vi "init.vi"(8 "error in":errorcluster, 10 "TBM module configuration in":refnum<class "TBM module configuration.lvclass">, 11 "bin datalogger runtime in":refnum<class "Binary datalogger runtime.lvclass">) -> (0 "error out":errorcluster, 1 "data allocations":T1, 2 "execution settings":T4, 3 "bin datalogger runtime out":refnum<class "Binary datalogger runtime.lvclass">)   [LabVIEW 2013, in "Binary datalogger runtime.lvclass"]
doc: "Provides an interface for initializing a module at runtime. While this interface performs no operations, a child should provide an override which may open any necessary references or sessions, allocate necessary memory, and perform any final configuration validataion before providing the full configuration <b>execution data</b> to the calling process."
uses:
  Binary datalogger runtime.lvclass
  <vilib>/NI/Tag Bus Module Framework/channel/TBM channel.lvclass
  <vilib>/NI/Tag Bus Module Framework/runtime/TBM module execution interface.lvclass
  configuration/Binary datalogger configuration.lvclass
  <vilib>/NI/Tag Bus Module Framework/runtime/execution settings.ctl
  control enum.ctl
  <vilib>/NI/Tag Bus/table/data table.ctl
  <vilib>/NI/Tag Bus/table/data table.lvlib
  <vilib>/NI/Tag Bus/dictionary/data dictionary.lvclass
  message to background process.ctl
  response enum.ctl
  response from background process.ctl
  <vilib>/NI/Tag Bus Module Framework/module configuration/TBM module configuration.lvclass
  <vilib>/NI/Tag Bus Module Framework/channel/data tables.ctl
  <vilib>/NI/Tag Bus/dictionary table pair.ctl
  <vilib>/NI/Tag Bus/tag bus.lvlib
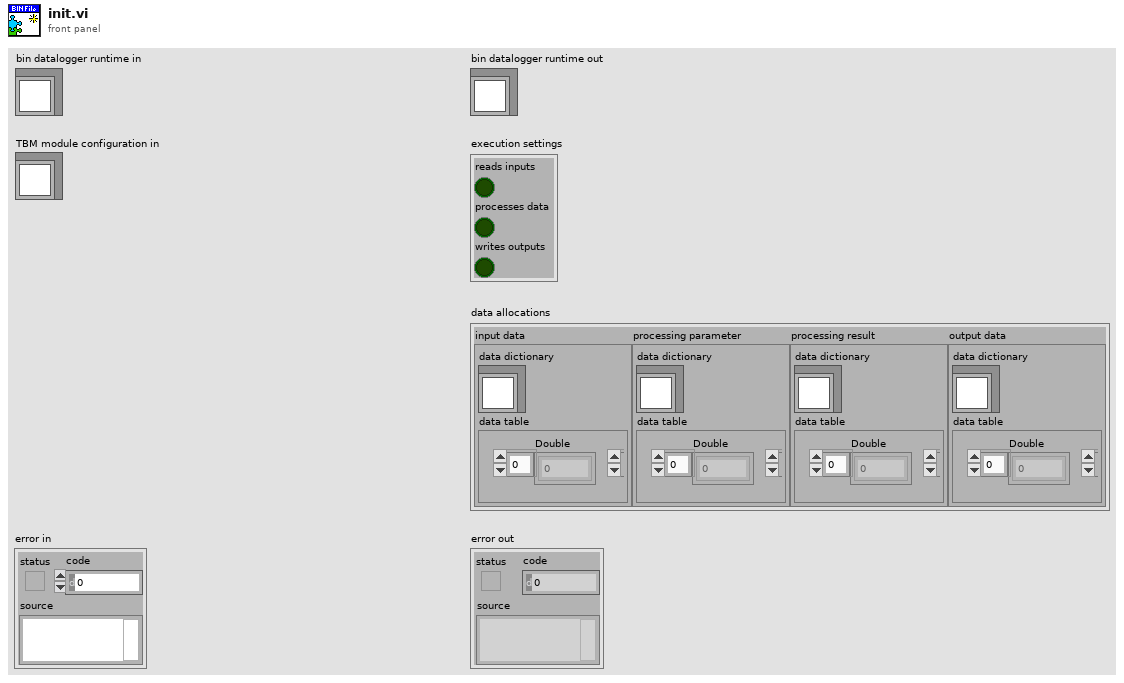
[diagram p1: front panel]
types:
  T1 = typedef "TBM channel.lvclass/data tables.ctl" = cluster{"input data":T2, "processing parameter":T2, "processing result":T2, "output data":T2}
  T2 = typedef "tag bus.lvlib/dictionary table pair.ctl" = cluster{"data dictionary":refnum<class "data dictionary.lvclass">, "data table":T3}
  T3 = typedef "tag bus.lvlib/data table.lvlib/data table.ctl" = cluster{"Double":dbl[], "Single":sgl[], "I64":i64[], "I32":i32[], "I16":i16[], "I8":i8[], "U64":u64[], "U32":u32[], "U16":u16[], "U8":u8[], "Boolean":bool[], "String":string[], "Array of Double":cluster{"DBL Array":dbl[]}[], "Array of Single":cluster{"SGL Array":sgl[]}[], "Array of I64":cluster{"I64 Array":i64[]}[], "Array of I32":cluster{"I32 Array":i32[]}[], "Array of I16":cluster{"I16 Array":i16[]}[], "Array of I8":cluster{"I8 Array":i8[]}[], "Array of U64":cluster{"U64 Array":u64[]}[], "Array of U32":cluster{"U32 Array":u32[]}[], "Array of U16":cluster{"U16 Array":u16[]}[], "Array of U8":cluster{"U8 Array":u8[]}[], "Array of Boolean":cluster{"Boolean Array":bool[]}[], "Array of String":cluster{"String Array":string[]}[]}
  T4 = typedef "TBM module execution interface.lvclass/execution settings.ctl" = cluster{"reads inputs":bool, "processes data":bool, "writes outputs":bool}
  T5 = cluster{"read mode":enum16{"polling", "blocking"}, "write mode":enum16{"polling", "blocking"}}
  T6 = typedef "Binary datalogger runtime.lvclass/response from background process.ctl" = cluster{"response enum":T7, "datapack":refnum<data-value>, "error code":i32}
  T7 = typedef "Binary datalogger runtime.lvclass/response enum.ctl" = enum16{"exit", "return buffer", "error"}
  T8 = typedef "Binary datalogger runtime.lvclass/message to background process.ctl" = cluster{"control enum":T9, "datapack":refnum<data-value>, "Time Stamp":timestamp}
  T9 = typedef "Binary datalogger runtime.lvclass/control enum.ctl" = enum16{"exit", "output data"}
  T10 = typedef "tag bus.lvlib/data dictionary.lvclass/full data dictionary.ctl" = cluster{"Double":string[], "Single":string[], "I64":string[], "I32":string[], "I16":string[], "I8":string[], "U64":string[], "U32":string[], "U16":string[], "U8":string[], "Boolean":string[], "String":string[], "Array of Double":string[], "Array of Single":string[], "Array of I64":string[], "Array of I32":string[], "Array of I16":string[], "Array of I8":string[], "Array of U64":string[], "Array of U32":string[], "Array of U16":string[], "Array of U8":string[], "Array of Boolean":string[], "Array of String":string[]}
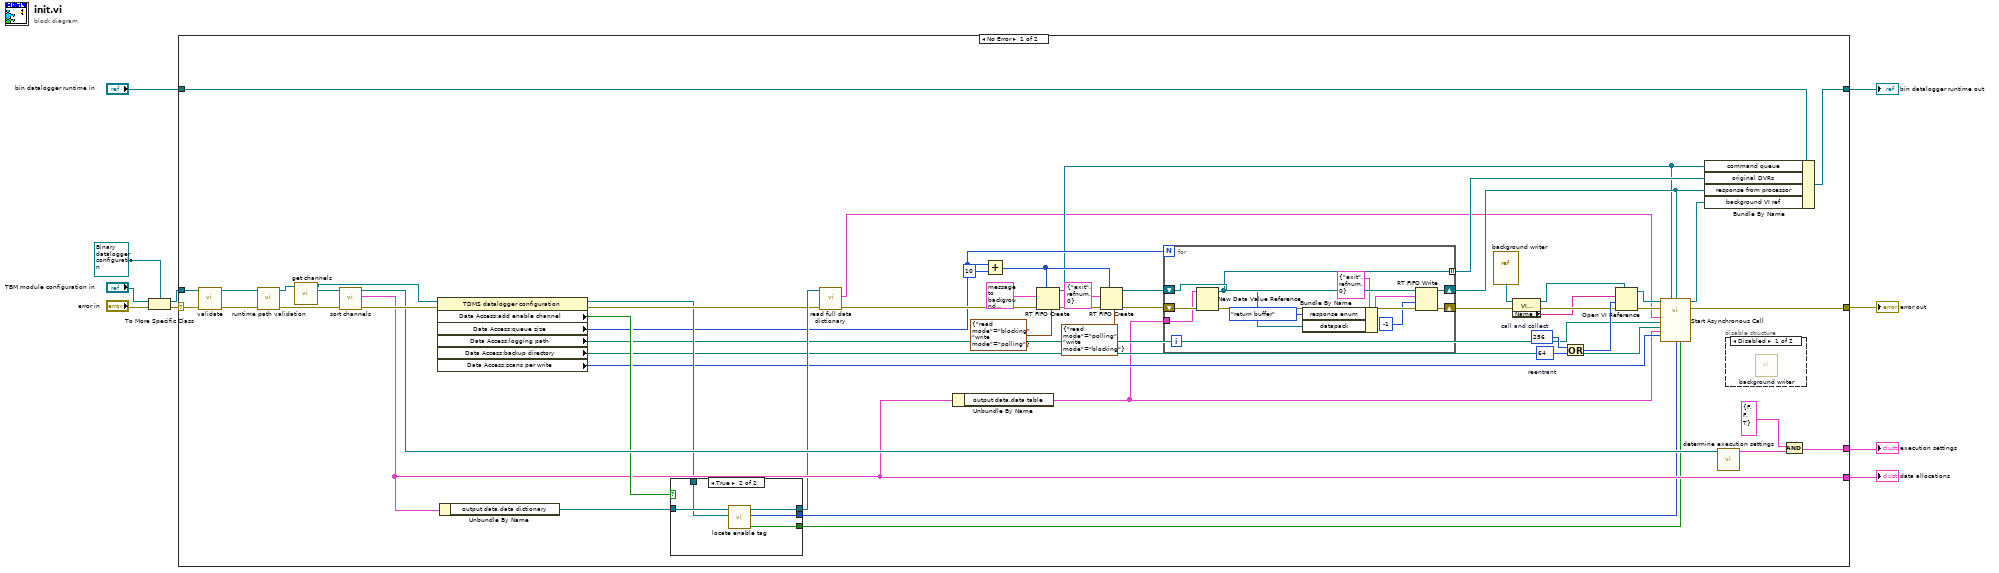
[diagram p0: block diagram]
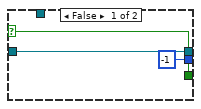
[diagram p2: hidden frame]
diagram:
  n1 = To More Specific Class(target class=refnum<class "Binary datalogger configuration.lvclass"> refnum ("Synchronous module configuration"), reference="TBM module configuration in", error in="error in") -> (specific class reference=w9:refnum<class "Binary datalogger configuration.lvclass">, error out=w10:errorcluster)
  n2 = case shown="No Error" w10 {
    selector: w10 -> [w60 w84]
    tunnel: w9 -> [w59 _]
    tunnel: "bin datalogger runtime in" -> [w58 w85]
    tunnel: [w57 w85] -> w4
    tunnel: [w47 w84] -> w3
    tunnel: [w44 _] -> w1
    tunnel: [w56 _] -> w2
    frame No Error {
      w52 = 64  # reentrant
      w51 = 256  # call and collect
      n3 = call-dynamic "validate.vi"("error in"=w60, "bin datalogger configuration in"=w59) -> ("error out"=w61:errorcluster, "bin datalogger configuration out"=w39:refnum<class "Binary datalogger configuration.lvclass">)  [unwired: 8 in]
      n4 = call "runtime path validation.vi"("error in"=w61, "bin datalogger configuration in"=w39) -> ("error out"=w40:errorcluster, "bin datalogger configuration out"=w38:refnum<class "Binary datalogger configuration.lvclass">)  [unwired: 8 in]
      n5 = call-dynamic "get channels.vi"("module configuration in"=w38) -> ("channels"=w36:refnum<class "TBM channel.lvclass">[], "module configuration out"=w37:refnum<class "Binary datalogger configuration.lvclass">)  [unwired: 9 in]
      n6 = call <vilib>:"sort channels.vi"("error in"=w40, "channels in"=w36) -> ("error out"=w64:errorcluster, "data allocations"=w44:T1, "channels out"=w62:refnum<class "TBM channel.lvclass">[])  [unwired: 7 in]
      n7 = property class="TDMS datalogger configuration"(reference=w37, error in=w64) -> (reference out=w33:refnum<class "Binary datalogger configuration.lvclass">, error out=w41:errorcluster, "Data Access:add enable channel"=w45:bool, "Data Access:queue size"=w25:u16, "Data Access:logging path"=w13:path, "Data Access:backup directory"=w12:path, "Data Access:scans per write"=w17:u16)
      n8 = Unbundle By Name(w44) -> ("output data.data dictionary"=w46:refnum<class "data dictionary.lvclass">)
      n9 = case shown="True" w45 {
        selector: w45 -> [w67 _]
        tunnel: w46 -> [w66 w72]
        tunnel: [w66 w71] -> w42
        tunnel: [w67 w69] -> w19
        tunnel: [-1 ("index") w70] -> w18
        tunnel: w33 -> [_ w68]
        frame False {
        }
        frame True {
          n10 = call "locate enable tag.vi"("bin datalogger configuration"=w68, "data dictionary in"=w72) -> ("found?"=w69:bool, "index"=w70:i32, "data dictionary out"=w71:refnum<class "data dictionary.lvclass">)  [unwired: 7 in]
        }
      }
      n11 = call <vilib>:"read full data dictionary.vi"("error in"=w41, "data dictionary in"=w42) -> ("error out"=w35:errorcluster, "dictionary"=w14:T10)  [unwired: 7 in, 1 out]
      n12 = Unbundle By Name(w44) -> ("output data.data table"=w11:T3)
      n13 = Add(x=w25, y=u16 10) -> (x+y=w23:u16)
      n14 = RT FIFO Create(1:T8 {"control enum"=enum."exit", "datapack"=refnum, "Time Stamp"=timestamp(0 s since 1904-01-01)} ("message"), 3:w35, 4:w23, 7:T5 {"read mode"=enum."blocking", "write mode"=enum."polling"} ("r/w modes (polling,polling)")) -> (8:w15:refnum<k33>, 11:w34:errorcluster)  [unwired: 4 in, 1 out]
      n15 = RT FIFO Create(1:T6 {"response enum"=enum."exit", "datapack"=refnum, "error code"=0} ("message"), 3:w34, 4:w23, 7:T5 {"read mode"=enum."polling", "write mode"=enum."blocking"} ("r/w modes (polling,polling)")) -> (8:w26:refnum<k33>, 11:w30:errorcluster)  [unwired: 4 in, 1 out]
      n16 = for {
        N: w25 -> [_]
        shift-right: [w80] -> w48
        shift-left: w30 -> [w83]
        tunnel: w11 -> [w82]
        tunnel: [w74] -> w27 mode=indexing
        shift-right: [w79] -> w16
        shift-left: w26 -> [w78]
        n17 = New Data Value Reference(data value=w82, error in=w83) -> (data value reference=w74:refnum<data-value>, error out=w81:errorcluster)
        n18 = Bundle By Name(cluster=T6 {"response enum"=enum."exit", "datapack"=refnum, "error code"=0} ("element"), "response enum"=response_enum."return buffer", "datapack"=w74) -> (w75:T6)
        n19 = RT FIFO Write(0:w78, 1:w75, 2:-1 ("timeout in ms (0)"), 3:w81) -> (8:w79:refnum<k33>, 11:w80:errorcluster)  [unwired: 1 in, 2 out]
      }
      n20 = vi-ref "background writer.vi"() -> (w22:refnum<vi>)
      n21 = property class="VI (strict)"(reference=w22, error in=w48) -> (reference out=w21:refnum<vi>, error out=w50:errorcluster, "Name"=w49:string)
      n22 = Or(x=w51, y=w52) -> (x .or. y?=w53:i32)
      n23 = Open VI Reference(type specifier VI Refnum (for type only)=w21, vi path=w49, options=w53, error in (no error)=w50) -> (vi reference=w20:refnum<vi>, error out=w54:errorcluster)  [unwired: 2 in]
      n24 = call-by-ref "Start Asynchronous Call"(reference=w20, error in=w54, "dictionary"=w14, "command queue"=w15, "response from processor"=w16, "logging path"=w13, "backup directory"=w12, "default data table"=w11, "scans per write"=w17, "enable channel (bool)"=w18, "has enable channel"=w19) -> (reference out=w43:refnum<vi>, error out=w47:errorcluster)  [unwired: 6 in, 1 out]
      n25 = Bundle By Name(cluster=w58, "command queue"=w15, "original DVRs"=w27, "response from processor"=w16, "background VI ref"=w43) -> (w57:refnum<class "Binary datalogger runtime.lvclass">)
      n26 = call <vilib>:"determine execution settings.vi"("channels"=w62) -> ("execution settings"=w63:T4)  [unwired: 10 in]
      n27 = disable-structure shown="Disabled" {
        frame Disabled {
          n28 = call "background writer.vi"() -> ()  [unwired: 15 in, 1 out]
        }
        frame Enabled {
        }
      }
      n29 = And(x=T4 {"reads inputs"=FALSE, "processes data"=FALSE, "writes outputs"=TRUE}, y=w63) -> (x .and. y?=w56:T4)
    }
    frame Error {
    }
  }
  "error out" <- w3
  "bin datalogger runtime out" <- w4
  "execution settings" <- w2
  "data allocations" <- w1
